vi "Load Config.vi"(8 "error in (no error)":errorcluster, 11 "DAQmxChannel in":refnum<class "DAQmxChannel.lvclass">) -> (0 "error out":errorcluster, 3 "DAQmxChannel out":refnum<class "DAQmxChannel.lvclass">)   [LabVIEW 2020, in "VolatusDAQConfig.lvlib" / "DAQmxChannel.lvclass"]
uses:
  DAQmxChannel.lvclass
  DAQmxChannel.lvclass/DAQmxChannel.ctl
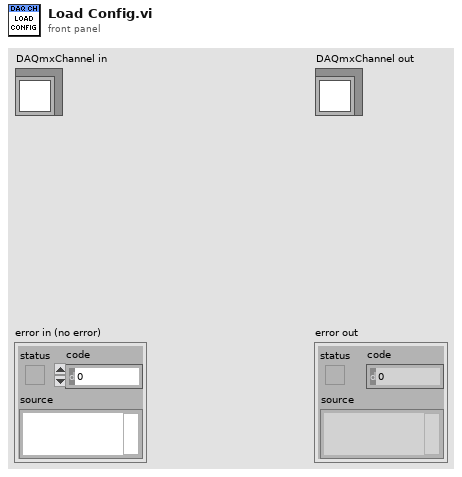
[diagram p1: front panel]
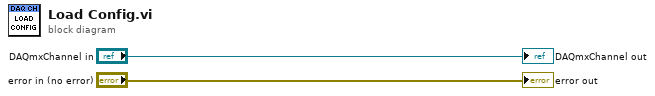
[diagram p0: block diagram]
diagram:
  "error out" <- "error in (no error)"
  "DAQmxChannel out" <- "DAQmxChannel in"
